vi "Remove Controls from List of Properties.vi"(11 "Data Cluster in":T1) -> (0 "Type of selection":T6(ring), 1 "Ctrl Tags":string[](array[string]), 3 "Data Cluster out":T1)   [LabVIEW 2020, in "Control Property Tree.lvlib"]
uses:
  Control Property Tree.lvlib
  Module Data--cluster.ctl
  Ctrl Properties Map Data.ctl
  Property array.ctl
  Selected Ctrls - List of Controls.ctl
  Selected Ctrls - List of Properties.ctl
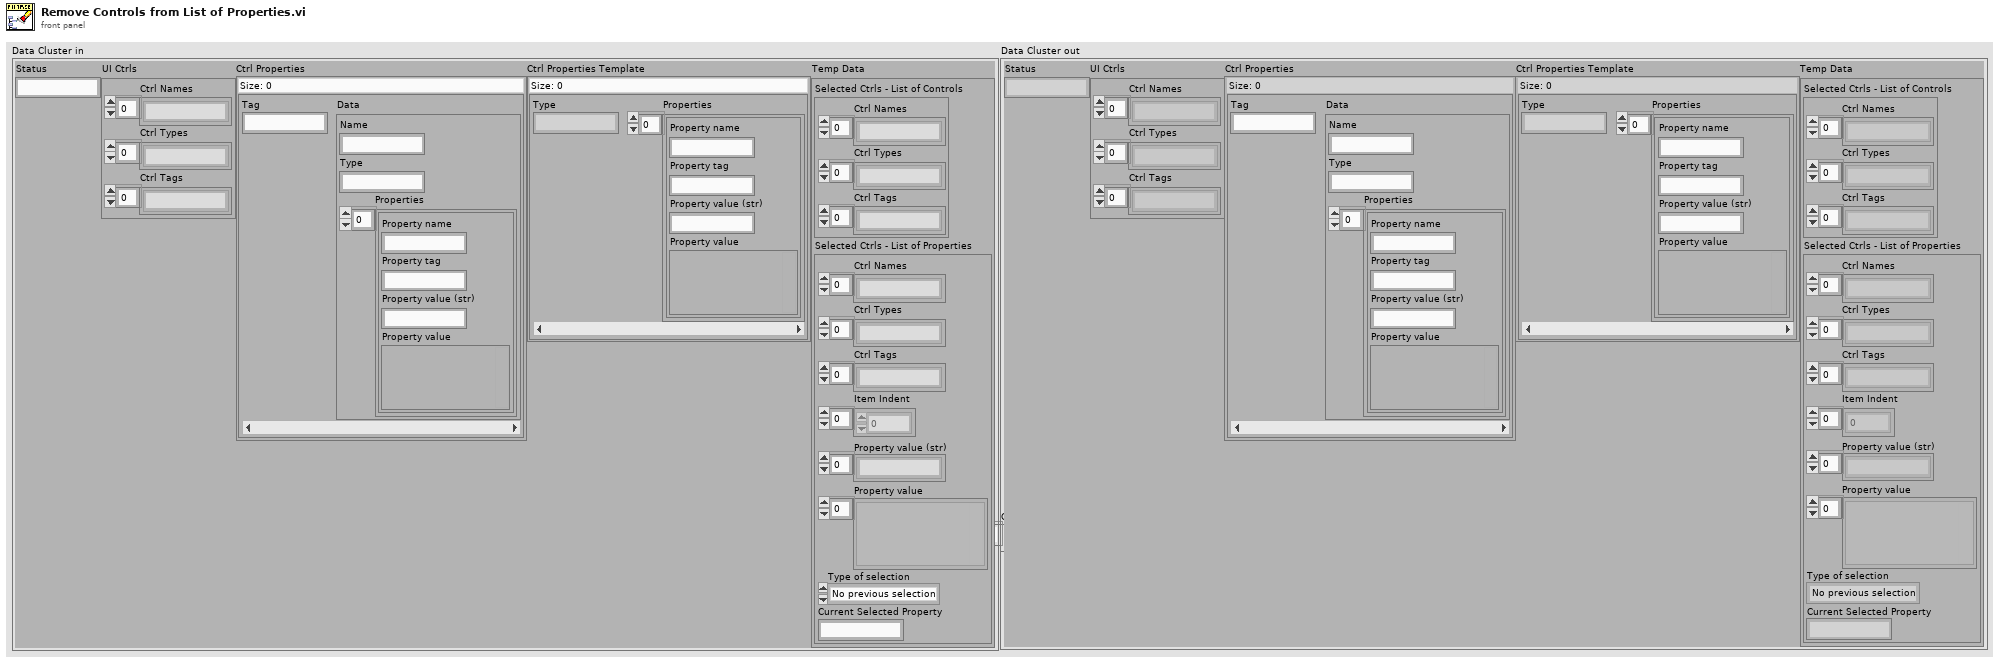
[diagram p1: front panel]
types:
  T1 = typedef "Control Property Tree.lvlib/Module Data--cluster.ctl" = cluster{"Status":string, "UI Ctrls":cluster{"Ctrl Names":string[], "Ctrl Types":string[], "Ctrl Tags":string[]}, "Ctrl Properties":map{string, T2}, "Ctrl Properties Template":map{string, T3}, "Temp Data":cluster{"Selected Ctrls - List of Controls":T4, "Selected Ctrls - List of Properties":T5}}
  T2 = typedef "Control Property Tree.lvlib/Ctrl Properties Map Data.ctl" = cluster{"Name":string, "Type":string, "Properties":T3}
  T3 = typedef "Control Property Tree.lvlib/Property array.ctl" = cluster{"Property name":string, "Property tag":string, "Property value (str)":string, "Property value":variant}[]
  T4 = typedef "Control Property Tree.lvlib/Selected Ctrls - List of Controls.ctl" = cluster{"Ctrl Names":string[], "Ctrl Types":string[], "Ctrl Tags":string[]}
  T5 = typedef "Control Property Tree.lvlib/Selected Ctrls - List of Properties.ctl" = cluster{"Ctrl Names":string[], "Ctrl Types":string[], "Ctrl Tags":string[], "Item Indent":i32[], "Property value (str)":string[], "Property value":variant[], "Type of selection":enum16{"No previous selection", "Control selected", "Property selected"}, "Current Selected Property":string}
  T6 = enum16{"No previous selection", "Control selected", "Property selected"}
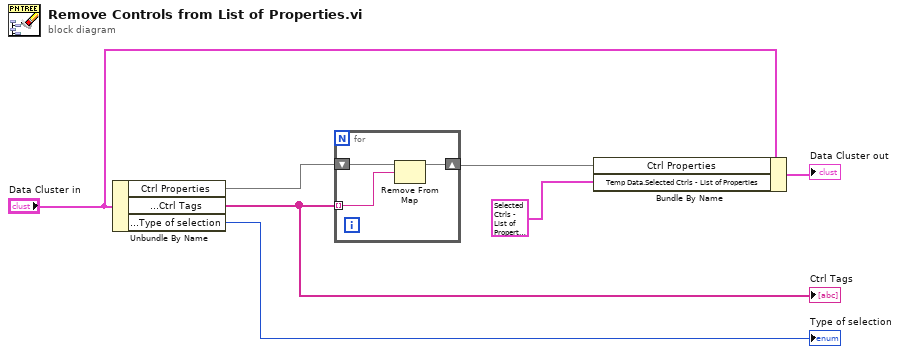
[diagram p0: block diagram]
diagram:
  n1 = Unbundle By Name("Data Cluster in") -> ("Ctrl Properties"=w6:map{string, T2}, "Temp Data.Selected Ctrls - List of Properties.Ctrl Tags"=w5:string[], "Temp Data.Selected Ctrls - List of Properties.Type of selection"=→"Type of selection":T6)
  "Ctrl Tags" <- w5
  n2 = for {
    tunnel: w5 -> [w9] mode=indexing
    shift-right: [w8] -> w4
    shift-left: w6 -> [w10]
    n3 = Remove From Map(10:w9, 11:w10) -> (3:w8:map{string, T2})  [unwired: 2 out]
  }
  n4 = Bundle By Name(cluster="Data Cluster in", "Ctrl Properties"=w4, "Temp Data.Selected Ctrls - List of Properties"=T5 {"Ctrl Names"=[], "Ctrl Types"=[], "Ctrl Tags"=[], "Item Indent"=[], "Property value (str)"=[], "Property value"=[], "Type of selection"=enum."No previous selection", "Current Selected Property"=""}) -> (→"Data Cluster out":T1)
